vi "SLSC Disable Buttons.vi"(8 "error in (no error)":errorcluster) -> (0 "error out":errorcluster)   [LabVIEW 2017, in "SLSC EDS System Explorer.lvlib"]
uses:
  System Explorer/SLSC EDS System Explorer.lvlib
  <vilib>/NI VeriStand/Custom Device API/Custom Device API.lvlib
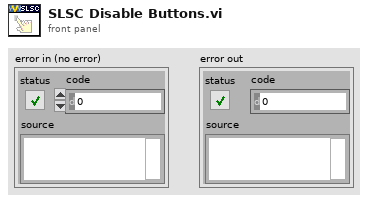
[diagram p1: front panel]
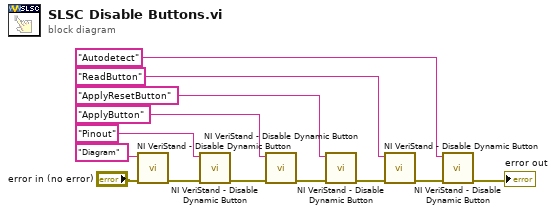
[diagram p0: block diagram]
diagram:
  n1 = call <vilib>:"NI VeriStand - Disable Dynamic Button.vi"("error in (no error)"="error in (no error)", "Button ID"="Diagram") -> ("error out"=w8:errorcluster)  [unwired: 9 in]
  n2 = call <vilib>:"NI VeriStand - Disable Dynamic Button.vi"("error in (no error)"=w8, "Button ID"="Pinout") -> ("error out"=w9:errorcluster)  [unwired: 9 in]
  n3 = call <vilib>:"NI VeriStand - Disable Dynamic Button.vi"("error in (no error)"=w9, "Button ID"="ApplyButton" ("x")) -> ("error out"=w6:errorcluster)  [unwired: 9 in]
  n4 = call <vilib>:"NI VeriStand - Disable Dynamic Button.vi"("error in (no error)"=w6, "Button ID"="ApplyResetButton" ("x")) -> ("error out"=w12:errorcluster)  [unwired: 9 in]
  n5 = call <vilib>:"NI VeriStand - Disable Dynamic Button.vi"("error in (no error)"=w12, "Button ID"="ReadButton" ("x")) -> ("error out"=w3:errorcluster)  [unwired: 9 in]
  n6 = call <vilib>:"NI VeriStand - Disable Dynamic Button.vi"("error in (no error)"=w3, "Button ID"="Autodetect" ("x")) -> ("error out"=→"error out":errorcluster)  [unwired: 9 in]
